vi "Get IPs and subnet masks.vi"(11 "error in (no error)":errorcluster) -> (4 "IP adresses":string[](array[string]), 6 "Subnets":string[](array[string]), 8 "Gateways":string[](array[string]), 10 "standard output":string, 15 "error out":errorcluster)   [LabVIEW 2020]
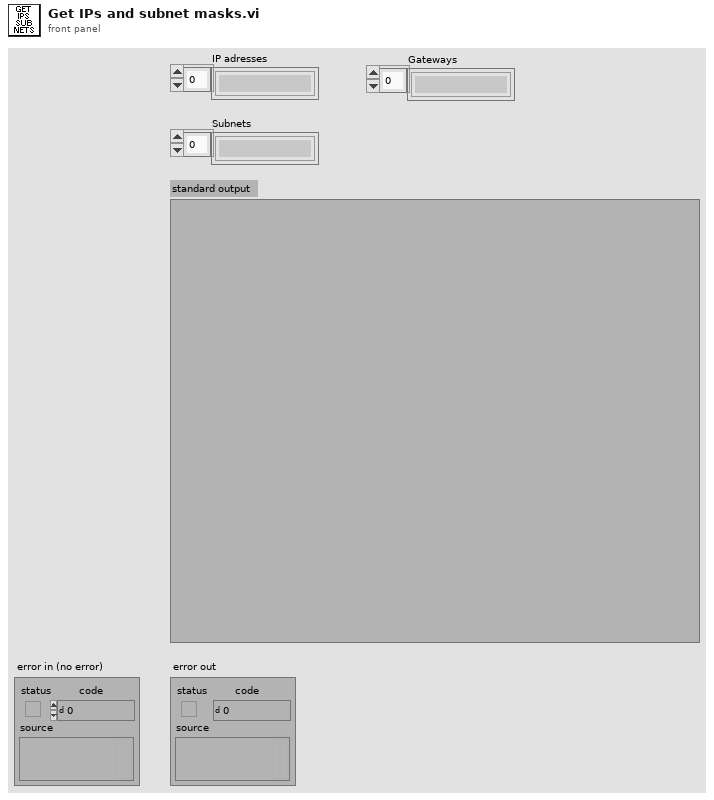
[diagram p1: front panel]
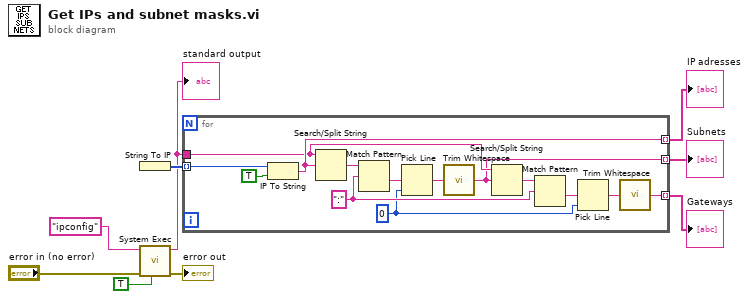
[diagram p0: block diagram]
diagram:
  n1 = String To IP() -> (0:w7:u32[])  [unwired: 1 in]
  n2 = call "System Exec.vi"("run minimized? (F)"=TRUE, "error in (no error)"="error in (no error)", "command line"="ipconfig") -> ("error out"=→"error out":errorcluster, "standard output"=w4:string)  [unwired: 5 in, 2 out]
  "standard output" <- w4
  n3 = for {
    tunnel: [w16] -> w8 mode=indexing
    tunnel: w4 -> [w17]
    tunnel: w7 -> [w19] mode=indexing
    tunnel: [w18] -> w9 mode=indexing
    tunnel: [w10] -> w1 mode=indexing
    w12 = 0 ("line index")
    w14 = ":" ("regular expression")
    n4 = IP To String(1:TRUE ("dot notation? (F)"), 2:w19) -> (0:w18:string)
    n5 = Search/Split String(string=w17, search string/char (-)=w18) -> (match + rest of string=w23:string)  [unwired: 1 in, 2 out]
    n6 = Match Pattern(string=w23, regular expression=w14) -> (after substring=w22:string)  [unwired: 1 in, 3 out]
    n7 = Pick Line(multi-line string=w22, line index=w12) -> (output string=w21:string)  [unwired: 1 in]
    n8 = call "Trim Whitespace.vi"("string"=w21) -> ("trimmed string"=w16:string)  [unwired: 1 in]
    n9 = Search/Split String(string=w17, search string/char (-)=w16) -> (match + rest of string=w15:string)  [unwired: 1 in, 2 out]
    n10 = Match Pattern(string=w15, regular expression=w14) -> (after substring=w13:string)  [unwired: 1 in, 3 out]
    n11 = Pick Line(multi-line string=w13, line index=w12) -> (output string=w11:string)  [unwired: 1 in]
    n12 = call "Trim Whitespace.vi"("string"=w11) -> ("trimmed string"=w10:string)  [unwired: 1 in]
  }
  "IP adresses" <- w9
  "Subnets" <- w8
  "Gateways" <- w1
